vi "Run All.vi"(8 "Error In":errorcluster) -> (0 "Error Out":errorcluster)   [LabVIEW 2018, in "Tests.lvlib" / "Readers.lvlib"]
uses:
  Readers.lvlib
  String/String.lvlib
  <vilib>/addons/_JKI Toolkits/Caraya/classes/Test/Test.lvclass
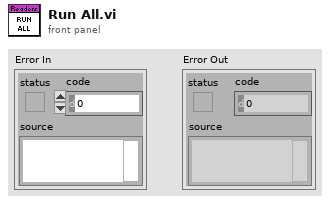
[diagram p1: front panel]
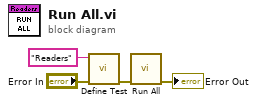
[diagram p0: block diagram]
diagram:
  n1 = call <vilib>:"Define Test.vi"("error in (no error)"="Error In", "Label (VI Title)"="Readers") -> ("error out"=w3:errorcluster)  [unwired: 9 in]
  n2 = call "Run All.vi"("Error In"=w3) -> ("Error Out"=→"Error Out":errorcluster)  [unwired: 10 in]
